vi "Configure Voltage.vi"(0 "VISA resource name":refnum<visa-resource-name>, 1 "Triggered Voltage Amplitude (1.0 V)":dbl=1.0 format="%#.4g", 2 "Voltage Slew Rate (9.9E+37 V)":dbl=9.9e+37 format="%#.4g", 5 "Voltage Range (300 V)":dbl=300.0 format="%#.4g", 7 "Voltage Amplitude (1.0 V)":dbl=1.0 format="%#.4g", 9 "Voltage Mode (0: Fix)":u16(ring) items=["Fixed", "Step", "Pulse", "List"], 11 "error in (no error)":errorcluster, 12 "Voltage Slew Mode (0: Fixed)":u16(ring) items=["Fixed", "Step", "Pulse", "List"], 13 "Triggered Voltage Slew Rate (9.9E+37 V)":dbl=9.9e+37 format="%#.4g") -> (4 "VISA resource name out":refnum<visa-resource-name>, 15 "error out":errorcluster)   [LabVIEW 2020, in "Agilent 681x Series.lvlib"]
doc: "Configures the voltage settings of the instrument."
uses:
  <instrlib>/Agilent 681x Series/Agilent 681x Series.lvlib
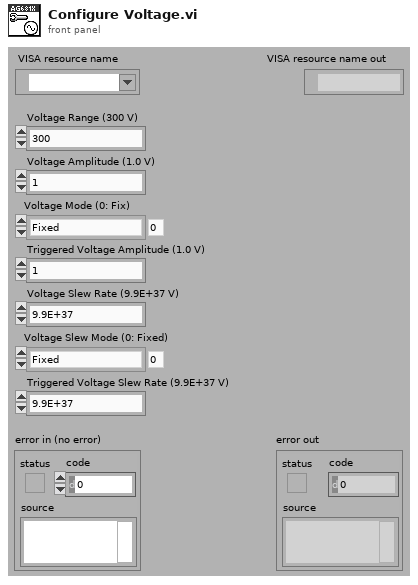
[diagram p1: front panel]
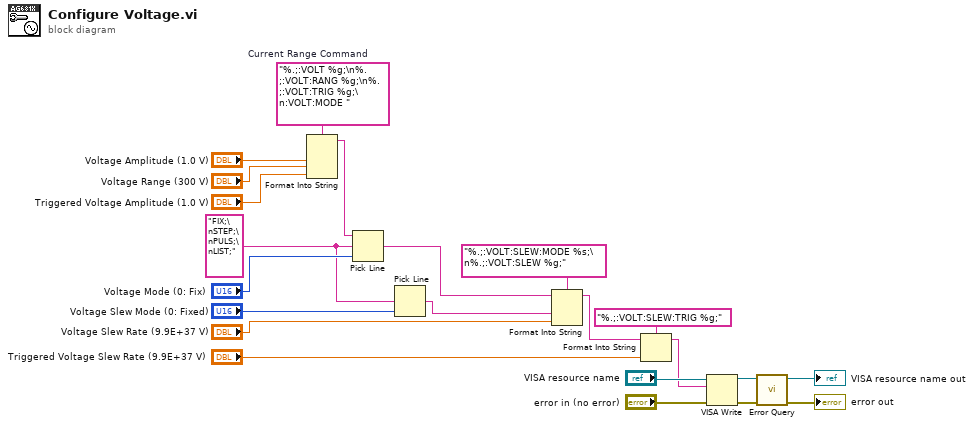
[diagram p0: block diagram]
diagram:
  w8 = "FIX;\nSTEP;\nPULS;\nLIST;" ("multi-line string")
  w18 = "%.;:VOLT %g;\n%.;:VOLT:RANG %g;\n%.;:VOLT:TRIG %g;\n:VOLT:MODE "  # Current Range Command
  n1 = Format Into String(format string=w18, "Voltage Amplitude (1.0 V)", "Voltage Range (300 V)", "Triggered Voltage Amplitude (1.0 V)") -> (resulting string=w15:string)  [unwired: 2 in, 1 out]
  n2 = Pick Line(string ("")=w15, multi-line string=w8, line index="Voltage Mode (0: Fix)") -> (output string=w6:string)
  n3 = Pick Line(multi-line string=w8, line index="Voltage Slew Mode (0: Fixed)") -> (output string=w9:string)  [unwired: 1 in]
  n4 = Format Into String(format string="%.;:VOLT:SLEW:MODE %s;\n%.;:VOLT:SLEW %g;", initial string=w6, w9, "Voltage Slew Rate (9.9E+37 V)") -> (resulting string=w3:string)  [unwired: 1 in, 1 out]
  n5 = Format Into String(format string="%.;:VOLT:SLEW:TRIG %g;", initial string=w3, "Triggered Voltage Slew Rate (9.9E+37 V)") -> (resulting string=w1:string)  [unwired: 1 in, 1 out]
  n6 = VISA Write(VISA resource name="VISA resource name", write buffer=w1, error in (no error)="error in (no error)") -> (VISA resource name out=w20:refnum<visa-resource-name>, error out=w19:errorcluster)  [unwired: 1 out]
  n7 = call <instrlib>:"Error Query.vi"("error in (no error)"=w19, "VISA resource name"=w20) -> ("error out"=→"error out":errorcluster, "VISA resource name out"=→"VISA resource name out":refnum<visa-resource-name>)  [unwired: 6 in, 2 out]
